vi "age364xa Set Voltage.vi"(0 "Output enabled (False)":bool=TRUE, 2 "error in (no error)":errorcluster, 3 "Voltage level (0.0 Volts)":dbl format="%.2p", 4 "Current limit (0 Amps)":dbl=0.5 format="%.2p", 5 "Instrument Resource Name (\"GPIB::5::INSTR\")":refnum<visa-resource-name>="GPIB::5::INSTR") -> (1 "error out":errorcluster)   [LabVIEW 2013]
doc: "DESCRIPTION:\nThis VI configures the HP E364XA power supplies to generate a DV voltage at the output.\n\nINSTRUCTIONS:\n1. Enter the resource name.\n2. Enter voltage level, current limit, OVP limit.\n3. Set output enabled switch to True if you want the generated voltage to appear at the instrument's output.\n4. Run the VI.\n\nNOTES:\nWhen this VI finishes, observe the over voltage protection status indicator. If the protection status is True, the instrument is in over voltage protection state and the instrument outputs zero voltage at this case.\n\nNotice the order of the hpe364xa component VIs in the block diagram. The first VI in a sequence is the hpe364xa Initialize.vi, which provides a VISA session to the instrument driver. The last VI in a sequence must be the hpe364xa Close.vi."
panel:
  in  "OVP limit (22.0 Volts)":dbl=22.0 format="%.2p"
  in  "OVP enabled (True)":bool
  # "© 2003, National Instruments, Corporation.  All Rights Reserved."
  # "For instructions,\nselect Show Context Help\nfrom the Help menu."
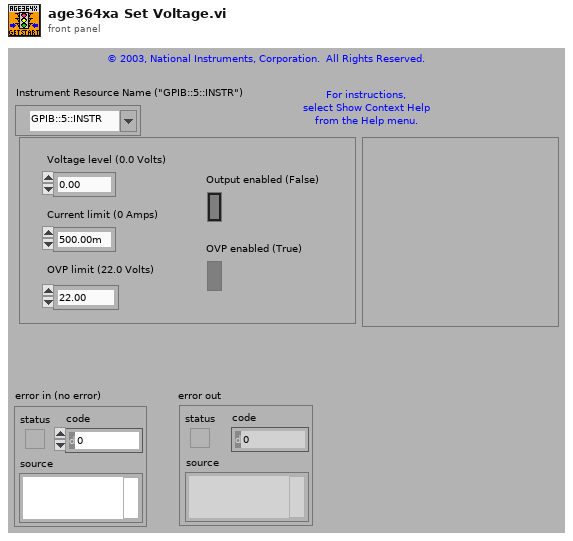
[diagram p1: front panel]
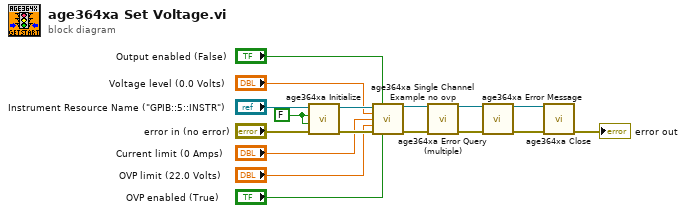
[diagram p0: block diagram]
diagram:
  w1 = FALSE ("Reset Device (T: Reset)")
  n1 = call <instrlib>:"age364xa Initialize.vi"("error in (no error)"="error in (no error)", "ID Query (T: Query)"=w1, "Reset Device (T: Reset)"=w1, "Instrument Resource Name"="Instrument Resource Name (\"GPIB::5::INSTR\")") -> ("error out"=w14:errorcluster, "dup VISA session"=w15:refnum<visa-resource-name>)  [unwired: 6 in]
  n2 = call "age364xa Single Channel Example no ovp.vi"("VISA session"=w15, "Output Enabled (False)"="Output enabled (False)", "Voltage Level (0.0 Volts)"="Voltage level (0.0 Volts)", "Current Limit (0 Amps)"="Current limit (0 Amps)", "OVP Limit (22.0 Volts)"="OVP limit (22.0 Volts)", "error in (no error)"=w14, "OVP Enabled (True)"="OVP enabled (True)") -> ("dup VISA session"=w8:refnum<visa-resource-name>, "error out"=w9:errorcluster)  [unwired: 7 in]
  n3 = call <instrlib>:"age364xa Error Query (multiple).vi"("error in (no error)"=w9, "VISA session"=w8) -> ("error out"=w10:errorcluster, "dup VISA session"=w11:refnum<visa-resource-name>)  [unwired: 6 in, 2 out]
  n4 = call <instrlib>:"age364xa Error Message.vi"("VISA session"=w11, "error in (no error)"=w10) -> ("dup VISA session"=w17:refnum<visa-resource-name>, "error out"=w16:errorcluster)  [unwired: 9 in, 3 out]
  n5 = call <instrlib>:"age364xa Close.vi"("error in (no error)"=w16, "VISA session"=w17) -> ("error out"=→"error out":errorcluster)  [unwired: 9 in]
